vi "ImportDatFile.vi"(8 "Error IN":errorcluster caption="에러 입력", 10 "FilePath":path, 11 "HEKAdat.lvclass IN":refnum<class "HEKAdat.lvclass">) -> (0 "Error OUT":errorcluster caption="에러 출력", 3 "HEKAdat.lvclass OUT":refnum<class "HEKAdat.lvclass">)   [LabVIEW 2017, in "HEKAdat.lvclass"]
uses:
  HEKAdat.lvclass
  HEKAdat.lvclass/HEKAdat.ctl
panel:
  out "String":string
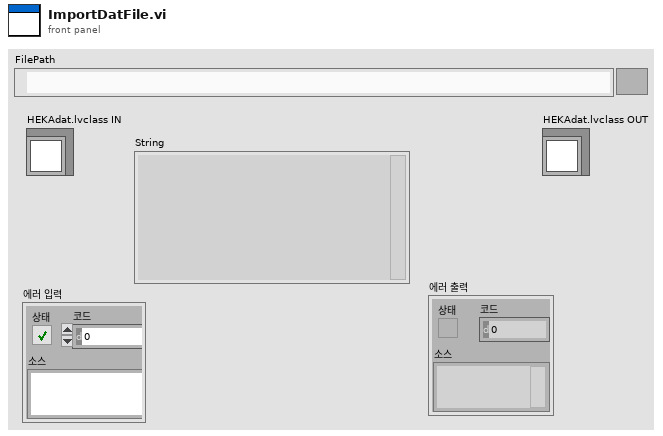
[diagram p1: front panel]
types:
  T1 = enum16{"big-endian, network order", "native, host order", "little-endian"}
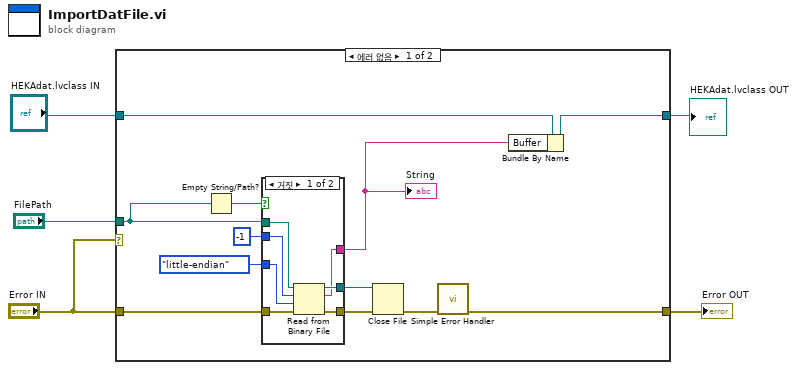
[diagram p0: block diagram]
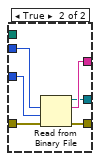
[diagram p2: hidden frame]
diagram:
  n1 = case shown="에러 없음" "Error IN" {
    tunnel: "Error IN" -> [w14 w31]
    tunnel: [w13 w31] -> w5
    tunnel: "HEKAdat.lvclass IN" -> [w9 w32]
    tunnel: [w7 w32] -> w3
    tunnel: "FilePath" -> [w6 _]
    frame No Error {
      n2 = Empty String/Path?(string/path=w6) -> (empty?=w11:bool)
      n3 = case shown="거짓" w11 {
        tunnel: T1."little-endian" ("바이트 순서(0:big-endian, network order)") -> [w24 w28]
        tunnel: [w23 w25] -> w10
        tunnel: [w22 w29] -> w16
        tunnel: w14 -> [w21 w30]
        tunnel: -1 ("numBytes") -> [w20 w27]
        tunnel: [w19 w26] -> w8
        tunnel: w6 -> [w18 _]
        frame False {
          n4 = Read from Binary File(8:w21, 9:w24, 10:w20, 11:w18) -> (0:w22:errorcluster, 2:w19:string, 3:w23:refnum<file>)  [unwired: 2 in, 1 out]
        }
        frame True {
          n5 = Read from Binary File(8:w30, 9:w28, 10:w27) -> (0:w29:errorcluster, 2:w26:string, 3:w25:refnum<file>)  [unwired: 3 in, 1 out]
        }
      }
      "String" <- w8
      n6 = Close File(refnum=w10, error in=w16) -> (error out=w15:errorcluster)  [unwired: 1 out]
      n7 = call <vilib>:"Simple Error Handler.vi"("error in (no error)"=w15) -> ("error out"=w13:errorcluster)  [unwired: 4 in, 4 out]
      n8 = Bundle By Name(cluster=w9, "Buffer"=w8) -> (w7:refnum<class "HEKAdat.lvclass">)
    }
    frame Error {
    }
  }
  "Error OUT" <- w5
  "HEKAdat.lvclass OUT" <- w3
